vi "Get Drive List.vi"(0 "error in (no error)":errorcluster) -> (2 "error out":errorcluster)   [LabVIEW 2011, in "API.lvlib"]
doc: "Uses an API call to retrieve a list of all available drives.\nThe output is an array of strings (one element for each drive letter)\nof the format \"c:\\\""
uses:
  API.lvlib
  kernel32.dll
panel:
  out "驱动器列表":string[](array[string])
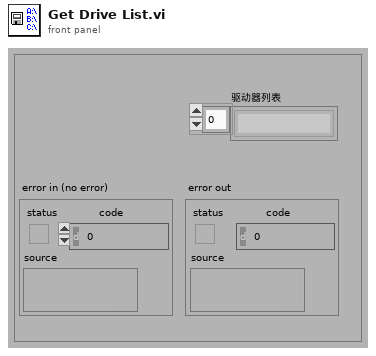
[diagram p1: front panel]
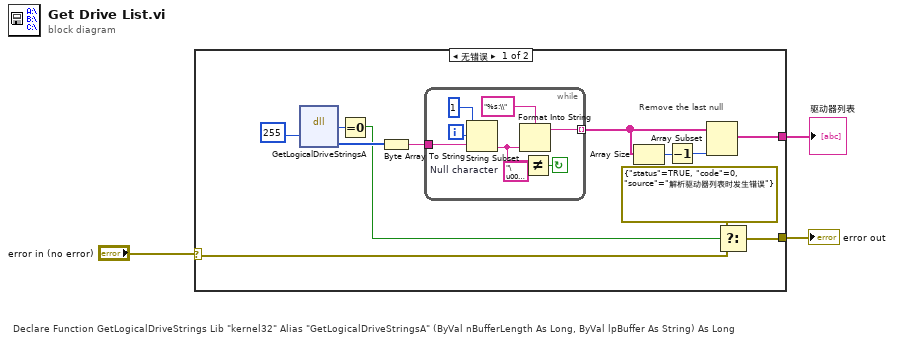
[diagram p0: block diagram]
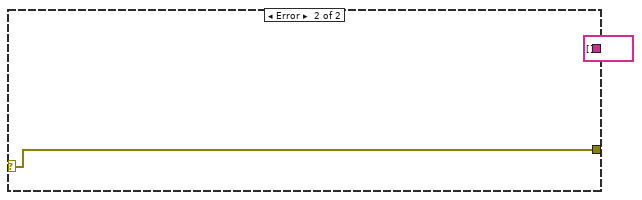
[diagram p2: hidden frame]
diagram:
  # "Declare Function GetLogicalDriveStrings Lib \"kernel32\" Alias \"GetLogicalDriveStringsA\" (ByVal nBufferLength As Long, ByVal lpBuffer As String) As Long"
  n1 = case shown="无错误" "error in (no error)" {
    selector: "error in (no error)" -> [w4 w24]
    tunnel: [w8 string[] []] -> w2
    tunnel: [w6 w24] -> w3
    frame No Error {
      # "Remove the last null"
      n2 = dll-call lib="kernel32.dll" fn="GetLogicalDriveStringsA" label="GetLogiicalDriveStrings"("nBufferLength"=255) -> ("返回类型"=w9:u32, "lpBuffer"=w13:i32[])  [unwired: 4 in, 3 out]
      n3 = Equal To 0?(x=w9) -> (x = 0?=w5:bool)
      n4 = Byte Array To String(unsigned byte array=w13) -> (string=w14:string)
      n5 = while "Iterate through the drives adding :\\" {
        tunnel: [w22] -> w12 mode=indexing
        tunnel: w14 -> [w19]
        i -> [w20]
        stop <- w16 continue-if-true
        w17 = "\u0000"  # Null character
        n6 = String Subset(string=w19, offset (0)=w20, length (rest)=1 ("length")) -> (substring=w18:string)
        n7 = Format Into String(format string="%s:\\", w18) -> (resulting string=w22:string)  [unwired: 2 in, 1 out]
        n8 = Not Equal?(x=w18, y=w17) -> (x != y?=w16:bool)
      }
      n9 = Array Size(array=w12) -> (size(s)=w11:i32)
      n10 = Decrement(x=w11) -> (x-1=w10:i32)
      n11 = Array Subset(array=w12, length=w10) -> (w8:string[])  [unwired: 1 in]
      n12 = Select(t=errorcluster {"status"=TRUE, "code"=0, "source"="解析驱动器列表时发生错误"} ("error in (no error)"), s=w5, f=w4) -> (s? t:f=w6:errorcluster)
    }
    frame Error {
    }
  }
  "error out" <- w3
  "驱动器列表" <- w2
